vi "execute.vi"(8 "error in (no error)":errorcluster, 9 "ImageAssembler in (B)":refnum<class "GenericComponent.lvclass">, 10 "ImagingMode in (A)":refnum<class "GenericComponent.lvclass">, 11 "AdapterMH110616ImagingModeToImageAssembler in":refnum<class "AdapterMH110616ImagingModeToImageAssembler.lvclass">) -> (0 "error out":errorcluster, 1 "ImageAssembler out (B)":refnum<class "GenericComponent.lvclass">, 2 "ImagingMode out (A)":refnum<class "GenericComponent.lvclass">, 3 "AdapterMH110616ImagingModeToImageAssembler out":refnum<class "AdapterMH110616ImagingModeToImageAssembler.lvclass">)   [LabVIEW 2010, in "AdapterMH110616ImagingModeToImageAssembler.lvclass"]
uses:
  AdapterMH110616ImagingModeToImageAssembler.lvclass
  common/classes/GenericComponent/GenericComponent/GenericComponent.lvclass
  ImagingMode/ImagingModeDL090130Frame/ImagingModeDL090130Frame/ImagingModeDL090130Frame.lvclass
  ImageAssembler/ImageAssemblerMG090623Binning/ImageAssemblerMG090623Binning/ImageAssemblerMG090623Binning.lvclass
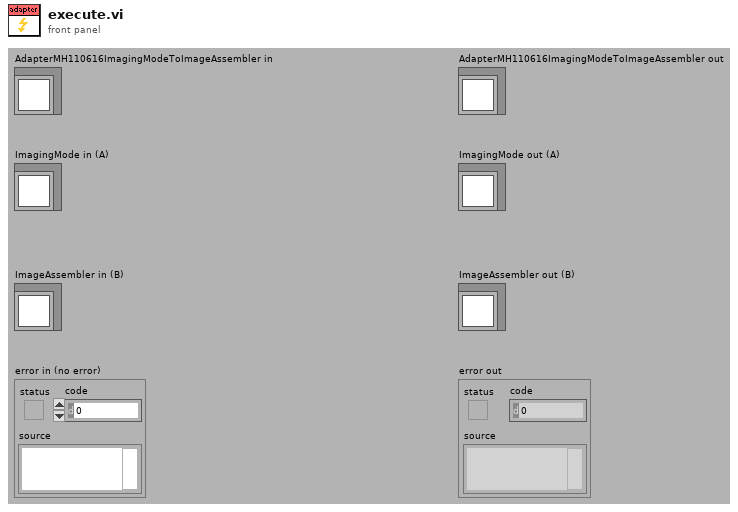
[diagram p1: front panel]
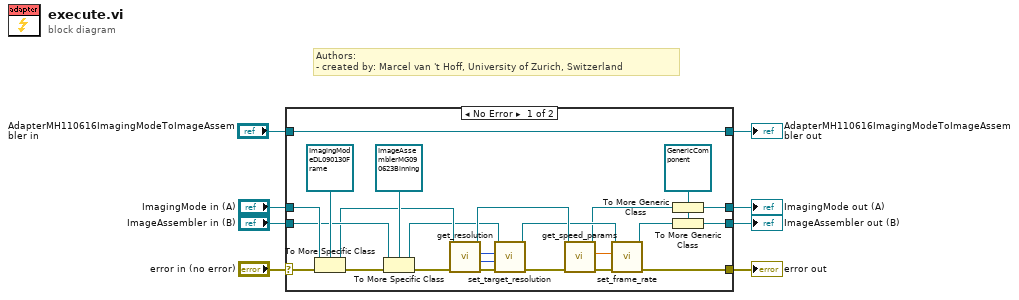
[diagram p0: block diagram]
diagram:
  # "Authors: \n- created by: Marcel van 't Hoff, University of Zurich, Switzerland"
  n1 = case shown="No Error" "error in (no error)" {
    selector: "error in (no error)" -> [w27 w36]
    tunnel: [w32 w35] -> w7
    tunnel: "AdapterMH110616ImagingModeToImageAssembler in" -> [w32 w35]
    tunnel: [w9 w36] -> w5
    tunnel: "ImagingMode in (A)" -> [w31 w34]
    tunnel: "ImageAssembler in (B)" -> [w29 w33]
    tunnel: [w12 w33] -> w2
    tunnel: [w11 w34] -> w1
    frame No Error {
      w16 = refnum<class "GenericComponent.lvclass"> refnum ("GenericComponent.lvclass")
      n2 = To More Specific Class(target class=refnum<class "ImagingModeDL090130Frame.lvclass"> refnum ("ImagingModeDL090130Frame.lvclass"), reference=w31, error in=w27) -> (specific class reference=w25:refnum<class "ImagingModeDL090130Frame.lvclass">, error out=w26:errorcluster)
      n3 = To More Specific Class(target class=refnum<class "ImageAssemblerMG090623Binning.lvclass"> refnum ("ImageAssemblerMG090623Binning.lvclass"), reference=w29, error in=w26) -> (specific class reference=w15:refnum<class "ImageAssemblerMG090623Binning.lvclass">, error out=w21:errorcluster)
      n4 = call-dynamic "get_resolution.vi"("error in (no error)"=w21, "ImagingModeDL090130Frame in"=w25) -> ("error out"=w22:errorcluster, "y resolution"=w23:i32, "x resolution"=w24:i32, "ImagingModeDL090130Frame out"=w20:refnum<class "ImagingModeDL090130Frame.lvclass">)  [unwired: 6 in]
      n5 = call-dynamic "set_target_resolution.vi"("error in (no error)"=w22, "y"=w23, "x"=w24, "MG090623BinningImageAssembler.lvclass in"=w15) -> ("error out"=w17:errorcluster, "MG090623BinningImageAssembler.lvclass out"=w14:refnum<class "ImageAssemblerMG090623Binning.lvclass">)  [unwired: 6 in]
      n6 = call-dynamic "get_speed_params.vi"("error in (no error)"=w17, "ImagingModeDL090130Frame in"=w20) -> ("error out"=w18:errorcluster, "frame rate"=w19:dbl[unit], "ImagingModeDL090130Frame out"=w10:refnum<class "ImagingModeDL090130Frame.lvclass">)  [unwired: 4 in, 3 out]
      n7 = call-dynamic "set_frame_rate.vi"("error in (no error)"=w18, "frame rate"=w19, "MG090623BinningImageAssembler.lvclass in"=w14) -> ("error out"=w9:errorcluster, "MG090623BinningImageAssembler.lvclass out"=w13:refnum<class "ImageAssemblerMG090623Binning.lvclass">)  [unwired: 7 in]
      n8 = To More Generic Class(target class=w16, reference=w10) -> (generic class reference=w11:refnum<class "GenericComponent.lvclass">)
      n9 = To More Generic Class(target class=w16, reference=w13) -> (generic class reference=w12:refnum<class "GenericComponent.lvclass">)
    }
    frame Error {
    }
  }
  "error out" <- w5
  "AdapterMH110616ImagingModeToImageAssembler out" <- w7
  "ImagingMode out (A)" <- w1
  "ImageAssembler out (B)" <- w2
